vi "vi_dll_close.vi"(10 "VI路径":path) -> ()   [LabVIEW 2018]
panel:
  out "错误输出":errorcluster
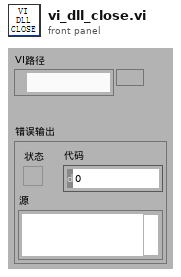
[diagram p1: front panel]
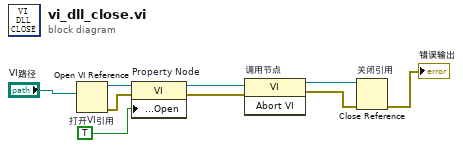
[diagram p0: block diagram]
diagram:
  n1 = Open VI Reference "打开VI引用"(vi path="VI路径") -> (vi reference=w9:refnum<vi>, error out=w6:errorcluster)  [unwired: 5 in]
  n2 = property on="Property Node" class="VI"(reference=w9, error in=w6, "Front Panel Window:Open"=TRUE ("结束前等待")) -> (reference out=w8:refnum<vi>, error out=w7:errorcluster)
  n3 = invoke on="调用节点" class="VI" method="Abort VI"(reference=w8, error in=w7) -> (reference out=w4:refnum<vi>, error out=w3:errorcluster)  [unwired: 1 in, 1 out]
  n4 = Close Reference "关闭引用"(reference=w4, error in (no error)=w3) -> (error out=→"错误输出":errorcluster)
